vi "BLOW.vi"(7 "arguments":string[](array[string]), 8 "dt":i32, 9 "Reinit":bool, 10 "bus_inputs":T1, 11 "bus_state":T2) -> (1 "Done":bool, 2 "bus_inputs out":T1, 3 "bus_state out":T2)   [LabVIEW 2013]
uses:
  roller/roller_des_state.ctl
  structures/bus_state_drivetrain.ctl
  structures/bus_state_collector.ctl
  structures/bus_state.ctl
  structures/bus_inputs.ctl
  collector/collector_shot_cal.ctl
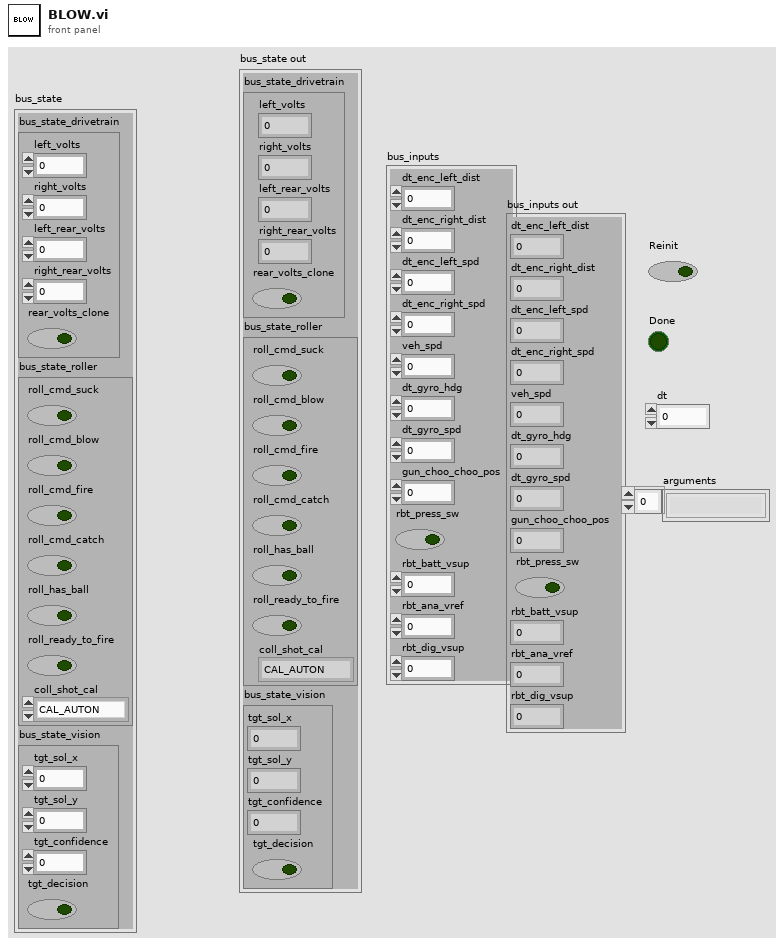
[diagram p1: front panel]
types:
  T1 = typedef "bus_inputs.ctl" = cluster{"dt_enc_left_dist":sgl, "dt_enc_right_dist":sgl, "dt_enc_left_spd":sgl, "dt_enc_right_spd":sgl, "veh_spd":sgl, "dt_gyro_hdg":sgl, "dt_gyro_spd":sgl, "gun_choo_choo_pos":sgl, "rbt_press_sw":bool, "rbt_batt_vsup":sgl, "rbt_ana_vref":dbl, "rbt_dig_vsup":dbl}
  T2 = typedef "bus_state.ctl" = cluster{"bus_state_drivetrain":T3, "bus_state_roller":T4, "bus_state_vision":cluster{"tgt_sol_x":dbl, "tgt_sol_y":dbl, "tgt_confidence":dbl, "tgt_decision":bool}}
  T3 = typedef "bus_state_drivetrain.ctl" = cluster{"left_volts":sgl, "right_volts":sgl, "left_rear_volts":sgl, "right_rear_volts":sgl, "rear_volts_clone":bool}
  T4 = typedef "bus_state_collector.ctl" = cluster{"roll_cmd_suck":bool, "roll_cmd_blow":bool, "roll_cmd_fire":bool, "roll_cmd_catch":bool, "roll_has_ball":bool, "roll_ready_to_fire":bool, "coll_shot_cal":T5}
  T5 = typedef "collector_shot_cal.ctl" = enum16{"CAL_AUTON", "CAL_CLOSE", "CAL_MID", "CAL_FAR"}
  T6 = typedef "roller_des_state.ctl" = enum16{"OFF", "SUCK", "BLOW"}
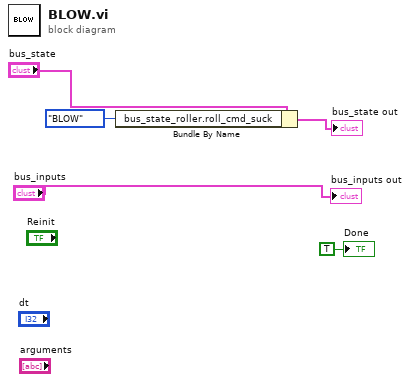
[diagram p0: block diagram]
diagram:
  n1 = Bundle By Name(cluster="bus_state", "bus_state_roller.roll_cmd_suck"=roller_des_state."BLOW" ("bus_state_roller.roller_des_state")) -> (→"bus_state out":T2)
  "bus_inputs out" <- "bus_inputs"
  "Done" <- TRUE ("Done")
